vi "CreateDataEvent.vi"(7 "Qbus":refnum<class "Qbus.lvclass">, 8 "error in (no error)":errorcluster, 9 "data":T1, 10 "Ir Data Event":T6, 11 "config in":T5) -> (0 "error out":errorcluster, 3 "config out":T5)   [LabVIEW 2017, in "IrDataEventCreator.lvlib"]
uses:
  <vilib>/addons/InsightCM/Devices/Shared/Ir/IrDataEventCreator/IrDataEventCreator.lvlib
  <vilib>/addons/InsightCM/Devices/Shared/Ir/IrDataEventCreator/controls/IrDataEvent.ctl
  <vilib>/addons/InsightCM/Devices/Shared/Common/DataEvent/controls/EventReference.ctl
  <vilib>/addons/InsightCM/Devices/Shared/Common/DataEvent/controls/Event.ctl
  <vilib>/addons/InsightCM/MessageBus/Base/controls/DataEvent.ctl
  <vilib>/addons/InsightCM/MessageBus/Base/controls/KeyValuePair.ctl
  <vilib>/addons/InsightCM/Devices/Shared/Common/DataEvent/controls/DataSet.ctl
  <vilib>/addons/InsightCM/MessageBus/Base/controls/DataSetMetadata.ctl
  <vilib>/addons/InsightCM/MessageBus/Base/controls/TrendPoint.ctl
  <vilib>/addons/InsightCM/MessageBus/Base/controls/TrendAlarmUpdate.ctl
  <vilib>/addons/InsightCM/MessageBus/Base/controls/TrendAlarmTransition.ctl
  <vilib>/addons/PointValueMap/controls/PointMap.ctl
  <vilib>/addons/InsightCM/Devices/Shared/Ir/IrDataEventCreator/controls/config.ctl
  <vilib>/addons/Qbus/Qbus.lvclass
  <vilib>/addons/InsightCM/Devices/Shared/Common/DataFlow/controls/Data.ctl
  <vilib>/addons/InsightCM/Utilities/DataAccessors/controls/wfmSGL_DVR.ctl
  <vilib>/addons/InsightCM/Devices/Shared/Common/DataFlow/controls/Type.ctl
  <vilib>/addons/InsightCM/Devices/Shared/Common/FileFlow/subVIs/GetFirstProcessModule_EventRef.vi
  <vilib>/addons/InsightCM/Devices/Shared/Common/FileFlow/FileFlow.lvlib
  <vilib>/addons/InsightCM/Devices/Shared/Common/DataEvent/DataEvent.lvlib
  <vilib>/addons/PointValueMap/PointValueMap.lvlib
  <vilib>/addons/InsightCM/Devices/Shared/Common/DataFlow/DataFlow.lvlib
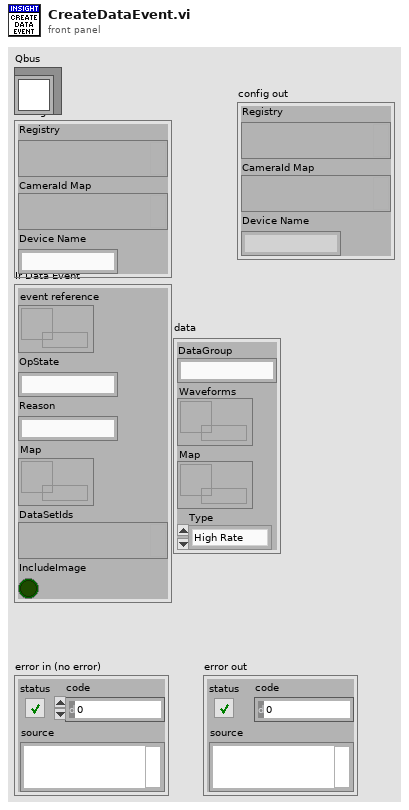
[diagram p1: front panel]
types:
  T1 = typedef "DataFlow.lvlib/Data.ctl" = cluster{"DataGroup":string, "Waveforms":T2, "Map":T3, "Type":T4}
  T2 = typedef "wfmSGL_DVR.ctl" = refnum<data-value>
  T3 = typedef "PointValueMap.lvlib/PointMap.ctl" = refnum<data-value>
  T4 = typedef "DataFlow.lvlib/Type.ctl" = enum16{"High Rate", "Low Rate", "Burst Mode"}
  T5 = typedef "IrDataEventCreator.lvlib/config.ctl" = cluster{"Registry":variant, "CameraId Map":variant, "Device Name":string}
  T6 = typedef "IrDataEventCreator.lvlib/IrDataEvent.ctl" = cluster{"event reference":T7, "OpState":string, "Reason":string, "Map":T3, "DataSetIds":variant, "IncludeImage":bool}
  T7 = typedef "DataEvent.lvlib/EventReference.ctl" = refnum<data-value>
  T8 = typedef "DataEvent.lvlib/Event.ctl" = cluster{"DataEvent":T9, "DataSets":T11[], "TrendPoints":T13[], "Alarms":T14[]}
  T9 = typedef "DataEvent.ctl" = cluster{"Id":string, "AssetNodeId":string, "Timestamp":i64, "Props":T10[]}
  T10 = typedef "KeyValuePair.ctl" = cluster{"Key":string, "Value":string}
  T11 = typedef "DataEvent.lvlib/DataSet.ctl" = cluster{"DataSetMetadata":T12, "Values":sgl[], "Values DVR":refnum<data-value>}
  T12 = typedef "DataSetMetadata.ctl" = cluster{"Id":string, "DataEventId":string, "AssetNodeId":string, "Type":string, "T0":i64, "Props":T10[]}
  T13 = typedef "TrendPoint.ctl" = cluster{"TrendPointId":string, "DataEventId":string, "Timestamp":i64, "Value":dbl, "Props":T10[]}
  T14 = typedef "TrendAlarmUpdate.ctl" = cluster{"RuleId":string, "Transition":T15}
  T15 = typedef "TrendAlarmTransition.ctl" = cluster{"At":i64, "Severity":i32, "Value":dbl}
  T16 = typedef "FileFlow.lvlib/data_eventRef.ctl" = cluster{"event reference":T7, "DataGroup":string, "OperatingState":string, "StreamId":string, "LastBlock":bool, "Map":T3, "TrendPoints Only":bool, "Extra Large File":bool}
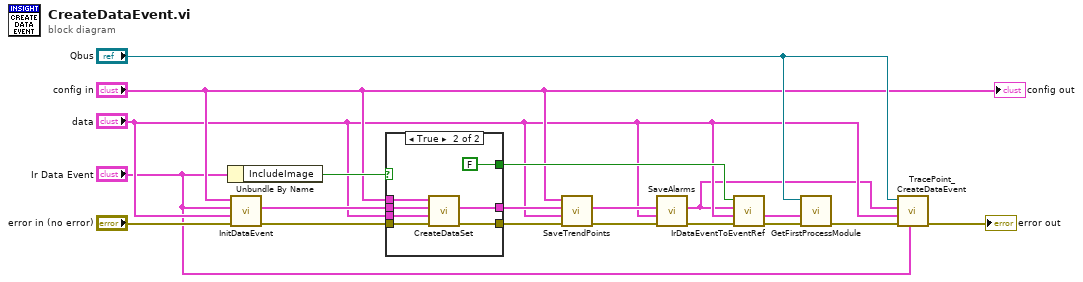
[diagram p0: block diagram]
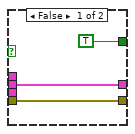
[diagram p2: hidden frame]
diagram:
  n1 = Unbundle By Name("Ir Data Event") -> ("IncludeImage"=w18:bool)
  n2 = call <vilib>:"InitDataEvent.vi"("error in (no error)"="error in (no error)", "data"="data", "Ir Data Event"="Ir Data Event", "config"="config in") -> ("error out"=w17:errorcluster, "data event"=w16:T8)  [unwired: 6 in]
  n3 = case shown="True" w18 {
    tunnel: w17 -> [w21 w29]
    tunnel: "data" -> [_ w28]
    tunnel: w16 -> [w22 w27]
    tunnel: [w22 w26] -> w8
    tunnel: [w21 w25] -> w7
    tunnel: "config in" -> [_ w24]
    tunnel: [TRUE ("TrendPoints Only") FALSE ("TrendPoints Only")] -> w13
    frame False {
    }
    frame True {
      n4 = call <vilib>:"CreateDataSet.vi"("error in (no error)"=w29, "data"=w28, "data event"=w27, "config in"=w24) -> ("error out"=w25:errorcluster, "data event out"=w26:T8)  [unwired: 6 in]
    }
  }
  n5 = call <vilib>:"SaveTrendPoints.vi"("error in (no error)"=w7, "data"="data", "data event in"=w8, "config in"="config in") -> ("error out"=w4:errorcluster, "data event out"=w6:T8)  [unwired: 6 in]
  n6 = call <vilib>:"SaveAlarms.vi"("error in (no error)"=w4, "data"="data", "data event in"=w6) -> ("error out"=w5:errorcluster, "data event out"=w1:T8)  [unwired: 7 in]
  n7 = call <vilib>:"IrDataEventToEventRef.vi"("error in (no error)"=w5, "data"="data", "data event in"=w1, "TrendPoints Only"=w13) -> ("error out"=w15:errorcluster, "file flow data"=w14:T16)  [unwired: 6 in]
  n8 = call-poly <vilib>:"GetFirstProcessModule.vi"("error in (no error)"=w15, "data"=w14, "Qbus in"="Qbus") -> ("error out"=w12:errorcluster)  [unwired: 7 in, 1 out]
  n9 = call <vilib>:"TracePoint_CreateDataEvent.vi"("Ir Data Event"="Ir Data Event", "error in (no error)"=w12, "data"="data", "data event"=w1, "Qbus"="Qbus") -> ("error out"=→"error out":errorcluster)  [unwired: 6 in]
  "config out" <- "config in"
